vi "DG535 Set Trigger Mode.vi"(6 "Relative to channel":T1, 7 "Output channel":T1, 8 "error in":errorcluster, 10 "Start delay":dbl format="%#_6ps", 11 "VISA resource name":refnum<visa-resource-name>) -> (0 "error out":errorcluster, 2 "Status byte":i32 format="%b", 3 "VISA resource name out":refnum<visa-resource-name>)   [LabVIEW 2020]
uses:
  DG Channel.ctl
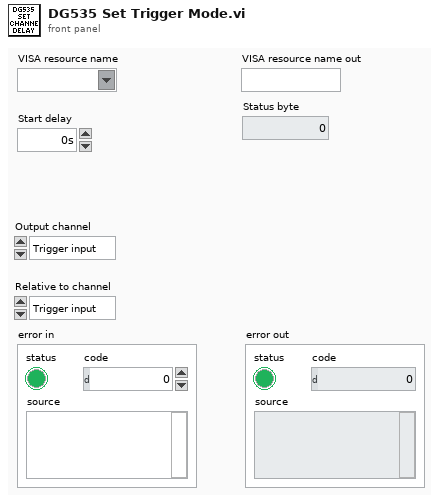
[diagram p1: front panel]
types:
  T1 = typedef "DG Channel.ctl" = enum16{"Trigger input", "T0", "A", "B", "AB", "C", "D", "CD"}
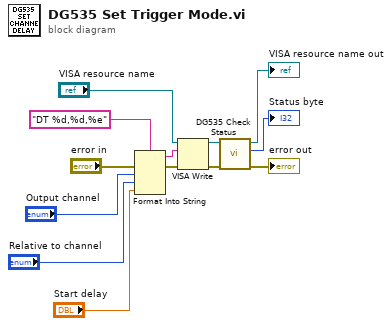
[diagram p0: block diagram]
diagram:
  n1 = Format Into String(format string="DT %d,%d,%e", error in="error in", "Output channel", "Relative to channel", "Start delay") -> (resulting string=w6:string, error out=w7:errorcluster)  [unwired: 1 in]
  n2 = VISA Write(VISA resource name="VISA resource name", write buffer=w6, error in (no error)=w7) -> (VISA resource name out=w3:refnum<visa-resource-name>, error out=w5:errorcluster)  [unwired: 1 out]
  n3 = call "DG535 Check Status.vi"("error in"=w5, "VISA resource name"=w3) -> ("error out"=→"error out":errorcluster, "Status byte"=→"Status byte":i32, "VISA resource name out"=→"VISA resource name out":refnum<visa-resource-name>)  [unwired: 7 in]
